vi "Antrenare neuroni ghicire cifre_litere_simboluri_grupuri de simboluri.vi"() -> ()   [LabVIEW 2025]
panel:
  out "Array":string[](array[string])=["1", "A", "#", ""]
  in  "Ce tip desenam?":enum16{"Cifre", "Litere", "Simboluri"}[](array[ring])=[enum."Cifre", enum."Litere", enum."Simboluri", enum."Cifre"]
  in  "Pixel patterns":bool[][](array[boolean])=[[FALSE, FALSE, FALSE, TRUE, FALSE, FALSE, FALSE, FALSE, FALSE, FALSE, TRUE, FALSE, FALSE, FALSE, FALSE, TRUE, FALSE, FALSE, FALSE, TRUE, FALSE, FALSE, FALSE, TRUE, TRUE, TRUE, FALSE, FALSE], [FALSE, FALSE, TRUE, TRUE, FALSE, FALSE, FALSE, FALSE, FALSE, TRUE, FALSE, TRUE, FALSE, FALSE, TRUE, TRUE, TRUE, TRUE, TRUE, TRUE, TRUE, FALSE, TRUE, FALSE, FALSE, FALSE, TRUE, FALSE], [FALSE, TRUE, FALSE, TRUE, FALSE, FALSE, FALSE, FALSE, TRUE, FALSE, FALSE, FALSE, TRUE, FALSE, FALSE, TRUE, FALSE, FALSE, FALSE, TRUE, FALSE, FALSE, TRUE, FALSE, FALSE, FALSE, TRUE, FALSE], [FALSE, FALSE, FALSE, TRUE, FALSE, FALSE, FALSE, FALSE, TRUE, FALSE, FALSE, FALSE, TRUE, FALSE, FALSE, TRUE, FALSE, FALSE, FALSE, TRUE, FALSE, FALSE, TRUE, FALSE, FALSE, FALSE, TRUE, FALSE], [FALSE, FALSE, FALSE, TRUE, FALSE, FALSE, FALSE, FALSE, TRUE, FALSE, FALSE, FALSE, TRUE, FALSE, FALSE, TRUE, FALSE, FALSE, FALSE, TRUE, FALSE, FALSE, FALSE, TRUE, TRUE, TRUE, FALSE, FALSE], [FALSE, FALSE, FALSE, TRUE, FALSE, FALSE, FALSE, FALSE, TRUE, TRUE, TRUE, TRUE, TRUE, FALSE, FALSE, TRUE, FALSE, FALSE, FALSE, TRUE, FALSE, FALSE, TRUE, FALSE, FALSE, FALSE, TRUE, FALSE], [FALSE, FALSE, FALSE, TRUE, FALSE, FALSE, FALSE, FALSE, TRUE, FALSE, FALSE, FALSE, TRUE, FALSE, FALSE, TRUE, FALSE, FALSE, FALSE, TRUE, FALSE, FALSE, TRUE, FALSE, FALSE, FALSE, TRUE, FALSE], [FALSE, FALSE, FALSE, TRUE, FALSE, FALSE, FALSE, FALSE, TRUE, FALSE, FALSE, FALSE, TRUE, FALSE, TRUE, TRUE, TRUE, TRUE, TRUE, TRUE, TRUE, FALSE, TRUE, FALSE, FALSE, FALSE, TRUE, FALSE], [FALSE, FALSE, TRUE, TRUE, TRUE, FALSE, FALSE, FALSE, TRUE, FALSE, FALSE, FALSE, TRUE, FALSE, FALSE, TRUE, FALSE, FALSE, FALSE, TRUE, FALSE, FALSE, FALSE, TRUE, TRUE, TRUE, FALSE, FALSE]]
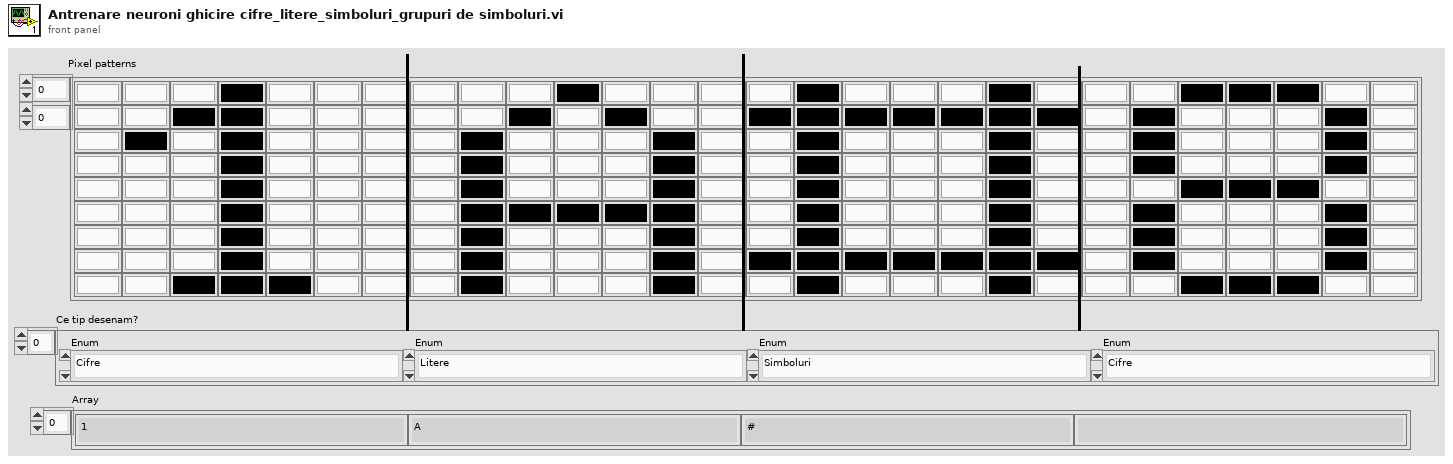
[diagram p1: front panel]
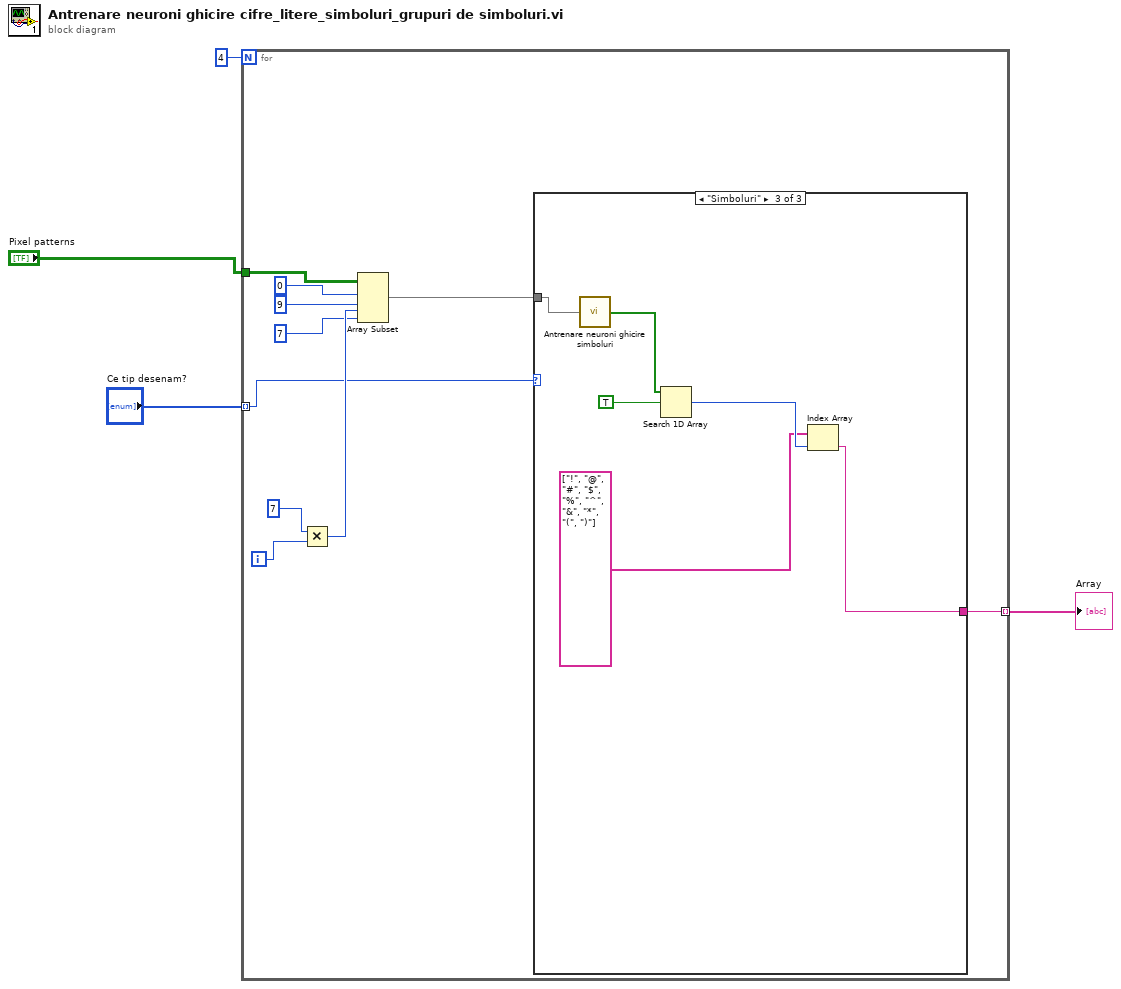
[diagram p0: block diagram]
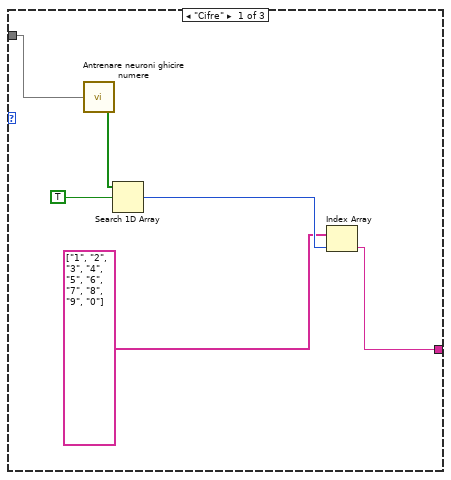
[diagram p2: hidden frame]
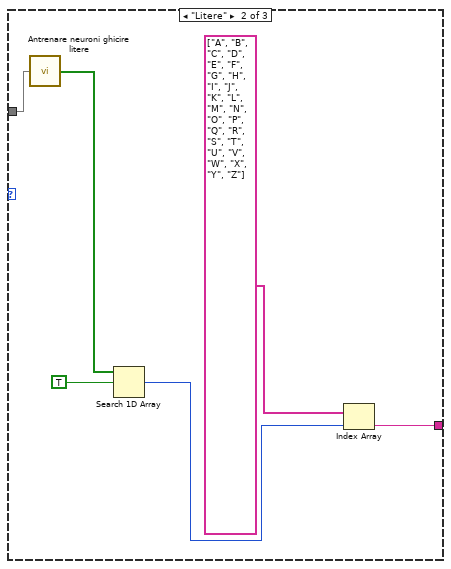
[diagram p3: hidden frame]
diagram:
  n1 = for {
    N: 4 -> [_]
    tunnel: "Pixel patterns" -> [w14]
    tunnel: "Ce tip desenam?" -> [w7] mode=indexing
    tunnel: [w5] -> w1 mode=indexing
    i -> [w13]
    n2 = Multiply(x=7, y=w13) -> (x*y=w9:i32)
    n3 = Array Subset "Array Subset"(array=w14, index (row)=0 ("index"), length (row)=9 ("length"), index (col)=w9, length (col)=7 ("length")) -> (w6:bool[][])
    n4 = case shown="\"Simboluri\"" w7 {
      tunnel: w6 -> [w20 w26 w32]
      tunnel: [w15 w21 w27] -> w5
      frame "Cifre" {
        n5 = call "Antrenare neuroni ghicire numere.vi"("Pixel patterns"=w20) -> ("Response"=w18:bool[])
        n6 = Search 1D Array(1D array=w18, element=TRUE) -> (index of element=w17:i32)  [unwired: 1 in]
        n7 = Index Array(array=string[] ["1", "2", "3", "4", "5", "6", "7", "8", "9", "0"], index=w17) -> (element=w15:string)
      }
      frame "Litere" {
        n8 = call "Antrenare neuroni ghicire litere.vi"("Pixel patterns"=w26) -> ("Response"=w25:bool[])
        n9 = Search 1D Array(1D array=w25, element=TRUE) -> (index of element=w22:i32)  [unwired: 1 in]
        n10 = Index Array(array=string[] ["A", "B", "C", "D", "E", "F", "G", "H", "I", "J", "K", "L", "M", "N", "O", "P", "Q", "R", "S", "T", "U", "V", "W", "X", "Y", "Z"], index=w22) -> (element=w21:string)
      }
      frame "Simboluri" {
        n11 = call "Antrenare neuroni ghicire simboluri.vi"("Pixel patterns"=w32) -> ("Response"=w30:bool[])
        n12 = Search 1D Array(1D array=w30, element=TRUE) -> (index of element=w29:i32)  [unwired: 1 in]
        n13 = Index Array(array=string[] ["!", "@", "#", "$", "%", "^", "&", "*", "(", ")"], index=w29) -> (element=w27:string)
      }
    }
  }
  "Array" <- w1
